vi "configuration_read.vi"(8 "error in (no error)":errorcluster, 11 "lv-builder-l3 in":refnum<class "lv-builder-l3.lvclass">) -> (0 "error out":errorcluster, 2 "configuration":variant, 3 "lv-builder-l3 out":refnum<class "lv-builder-l3.lvclass">)   [LabVIEW 2015, in "lv-builder-l3.lvlib" / "lv-builder-l3.lvclass"]
uses:
  lv-builder-l3.lvclass
  lv-builder-l3.lvclass/lv-builder-l3.ctl
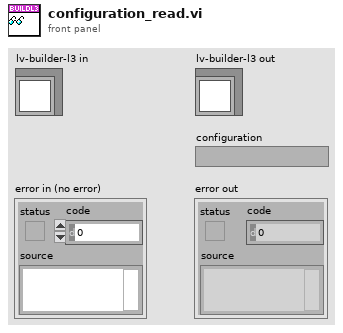
[diagram p1: front panel]
types:
  T1 = typedef "lv-builder-l3.lvlib/configuration.ctl" = cluster{"l3_archive_file_path":string}
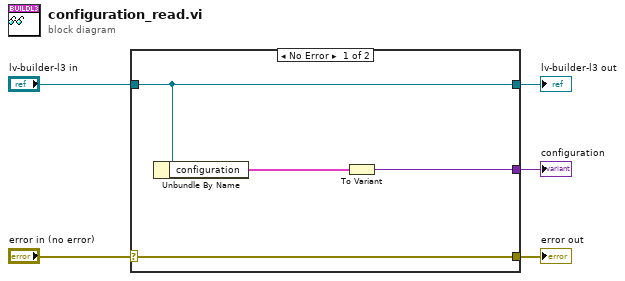
[diagram p0: block diagram]
diagram:
  n1 = case shown="No Error" "error in (no error)" {
    selector: "error in (no error)" -> [w9 w10]
    tunnel: [w9 w10] -> w4
    tunnel: [w8 w11] -> w2
    tunnel: "lv-builder-l3 in" -> [w8 w11]
    tunnel: [w6 _] -> w1
    frame No Error {
      n2 = Unbundle By Name(w8) -> ("configuration"=w7:T1)
      n3 = To Variant(anything=w7) -> (Variant=w6:variant)
    }
    frame Error {
    }
  }
  "error out" <- w4
  "lv-builder-l3 out" <- w2
  "configuration" <- w1
